vi "produceTriggerTick.vi"(8 "error in (no error)":errorcluster, 10 "Channel":refnum<class "Channel.lvclass">, 11 "ScriptEvent in":refnum<class "ScriptEvent.lvclass">) -> (0 "error out":errorcluster, 2 "timingTick":refnum<class "ScriptEventList.lvclass">, 3 "ScriptEvent out":refnum<class "ScriptEvent.lvclass">)   [LabVIEW 2011, in "Tools.lvlib" / "Scripting.lvlib" / "ScriptEvent.lvclass"]
uses:
  ScriptEvent.lvclass
  DatabaseHelpers/Database Objects/Channel/Channel.lvclass
  ScriptEventList/ScriptEventList.lvclass
  ScriptEvent.lvclass/ScriptEvent.ctl
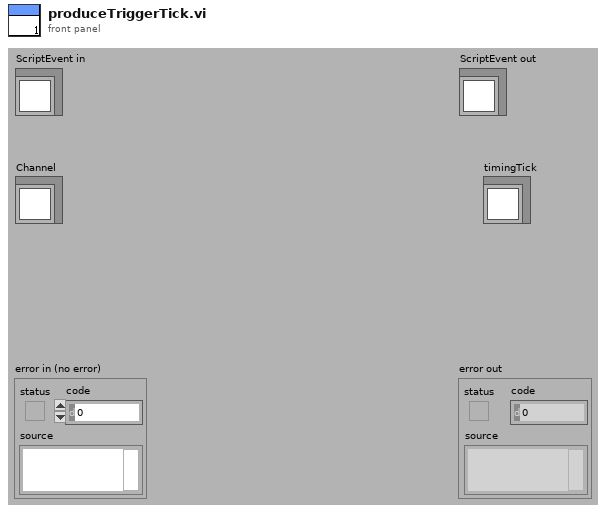
[diagram p1: front panel]
types:
  T1 = enum16{"changeValue", "pulse", "clock", "rampUp", "rampDown", "singleTone", "singleToneRamp", "playFile"}
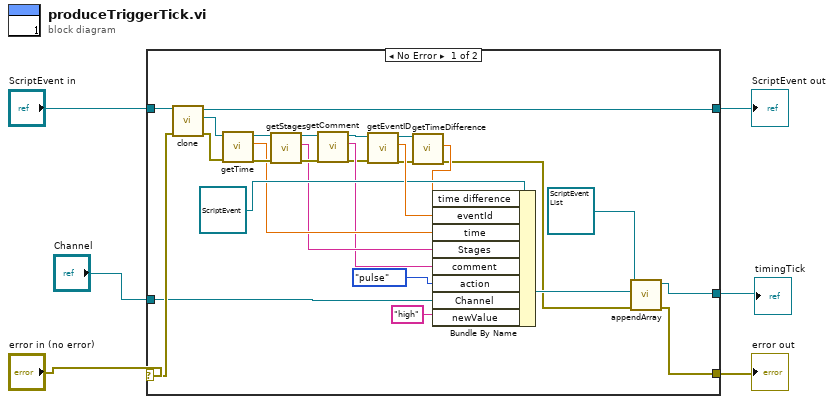
[diagram p0: block diagram]
diagram:
  n1 = case shown="No Error" "error in (no error)" {
    selector: "error in (no error)" -> [w26 w35]
    tunnel: [w29 w35] -> w3
    tunnel: [w27 w34] -> w5
    tunnel: "ScriptEvent in" -> [w28 w34]
    tunnel: [w31 _] -> w1
    tunnel: "Channel" -> [w25 _]
    frame No Error {
      n2 = call-dynamic "clone.vi"("error in (no error)"=w26, "ScriptEvent in"=w28) -> ("error out"=w22:errorcluster, "clone"=w23:refnum<class "ScriptEvent.lvclass">, "ScriptEvent out"=w27:refnum<class "ScriptEvent.lvclass">)  [unwired: 7 in]
      n3 = call "getTime.vi"("error in (no error)"=w22, "ScriptEvent.lvclass in"=w23) -> ("error out"=w21:errorcluster, "time"=w14:dbl, "ScriptEvent.lvclass out"=w20:refnum<class "ScriptEvent.lvclass">)  [unwired: 7 in]
      n4 = call "getStages.vi"("error in (no error)"=w21, "ScriptEvent.lvclass in"=w20) -> ("error out"=w19:errorcluster, "Stage"=w13:string, "ScriptEvent.lvclass out"=w18:refnum<class "ScriptEvent.lvclass">)  [unwired: 7 in]
      n5 = call "getComment.vi"("error in (no error)"=w19, "ScriptEvent.lvclass in"=w18) -> ("error out"=w11:errorcluster, "comment"=w12:string, "ScriptEvent.lvclass out"=w16:refnum<class "ScriptEvent.lvclass">)  [unwired: 7 in]
      n6 = call "getEventID.vi"("error in (no error)"=w11, "ScriptEvent in"=w16) -> ("error out"=w10:errorcluster, "eventId"=w17:dbl, "ScriptEvent out"=w9:refnum<class "ScriptEvent.lvclass">)  [unwired: 7 in]
      n7 = call "getTimeDifference.vi"("error in (no error)"=w10, "ScriptEvent.lvclass in"=w9) -> ("error out"=w7:errorcluster, "time difference"=w8:dbl)  [unwired: 7 in, 1 out]
      n8 = Bundle By Name(cluster=refnum<class "ScriptEvent.lvclass"> refnum ("Tools.lvlib:Scripting.lvlib:ScriptEvent.lvclass"), "time difference"=w8, "eventId"=w17, "time"=w14, "Stages"=w13, "comment"=w12, "action"=T1."pulse", "Channel"=w25, "newValue"="high") -> (w32:refnum<class "ScriptEvent.lvclass">)
      n9 = call "appendArray.vi"("error in (no error)"=w7, "ScriptEvent"=w32, "ScriptEventList in"=refnum<class "ScriptEventList.lvclass"> refnum) -> ("error out"=w29:errorcluster, "ScriptEventList out"=w31:refnum<class "ScriptEventList.lvclass">)  [unwired: 6 in, 1 out]
    }
    frame Error {
    }
  }
  "error out" <- w3
  "ScriptEvent out" <- w5
  "timingTick" <- w1
